vi "Get Image HSV Data.vi"(11 "image data":T1) -> (3 "HSV[]":T2(array[cluster]))   [LabVIEW 2014, in "HSV Distance Comparison.lvclass"]
uses:
  HSV Distance Comparison.lvclass
  <vilib>/picture/picture.llb/imagedata.ctl
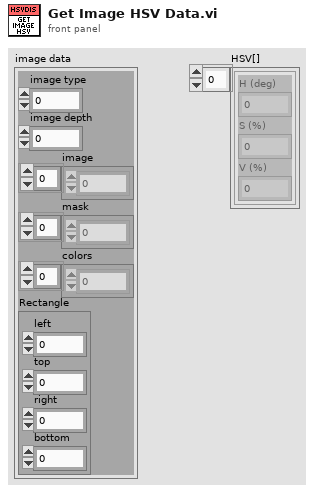
[diagram p1: front panel]
types:
  T1 = typedef "imagedata.ctl" = cluster{"image type":i32, "image depth":i32, "image":u8[], "mask":u8[], "colors":u32[], "Rectangle":cluster{"left":i16, "top":i16, "right":i16, "bottom":i16}}
  T2 = cluster{"H (deg)":dbl, "S (%)":dbl, "V (%)":dbl}[]
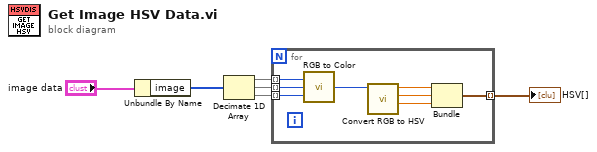
[diagram p0: block diagram]
diagram:
  n1 = Unbundle By Name("image data") -> ("image"=w2:u8[])
  n2 = Decimate 1D Array(w2) -> (w3:u8[], w4:u8[], w5:u8[])
  n3 = for {
    tunnel: w3 -> [w14] mode=indexing
    tunnel: w4 -> [w13] mode=indexing
    tunnel: w5 -> [w12] mode=indexing
    tunnel: [w7] -> w6 mode=indexing
    n4 = call <vilib>:"RGB to Color.vi"("B"=w12, "G"=w13, "R"=w14) -> ("Color"=w11:u32)
    n5 = call "Convert RGB to HSV.vi"("Color Box"=w11) -> ("V (%)"=w8:dbl, "S (%)"=w9:dbl, "H (deg)"=w10:dbl)  [unwired: 8 in]
    n6 = Bundle("H (deg)"=w10, "S (%)"=w9, "V (%)"=w8) -> (w7:cluster{"H (deg)":dbl, "S (%)":dbl, "V (%)":dbl})  [unwired: 1 in]
  }
  "HSV[]" <- w6
